vi "DetectHardware.vi"(8 "error in (no error)":errorcluster, 11 "Microscope_RM21 in":refnum<class "Microscope_RM21.lvclass">) -> (0 "error out":errorcluster, 3 "Microscope_RM21 out":refnum<class "Microscope_RM21.lvclass">)   [LabVIEW 2020, in "Microscope_RM21.lvlib" / "Microscope_RM21.lvclass"]
uses:
  Microscope_RM21.lvclass
  D:/Daguan/Development/MMicroscopyFramework/Model/Hardware Abstraction Layer/Microscope/Microscope/Microscope.lvclass
  Stage_MadCityLab/Stage_MadCityLab/Stage_MadCityLab.lvclass
  D:/Daguan/Development/MMicroscopyFramework/Model/Hardware Abstraction Layer/Component/Device/Device/Device.lvclass
  Stage_MadCityLabMicro/Stage_MadCityLabMicro/Stage_MadCityLabMicro.lvclass
  DAQ_QPT_Throlab/DAQ_QPT_Throlab/DAQ_QPT_Throlab.lvclass
  Camera_Prime95B/Camera_Prime95B/Camera_Prime95B.lvclass
  Laser_Oxxius/Laser_Oxxius/Laser_Oxxius.lvclass
  Hardware Abstraction Layer/Microscope/Microscope/Microscope.lvclass
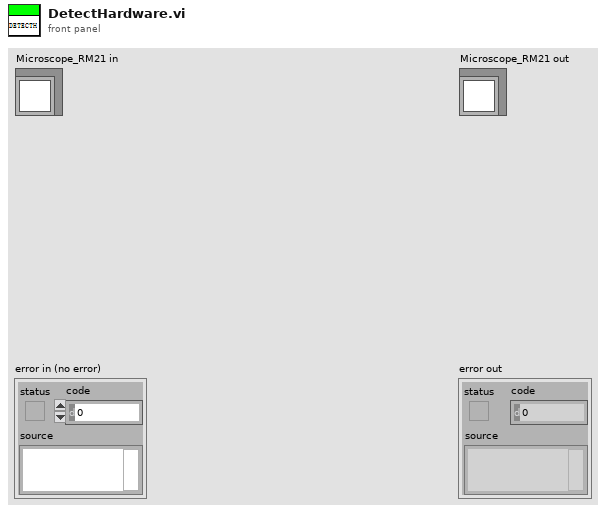
[diagram p1: front panel]
types:
  T1 = cluster{"Label":string, "DeviceType":string, "DefaultDevice? (F)":bool, "StartAcquiring? (F)":bool}
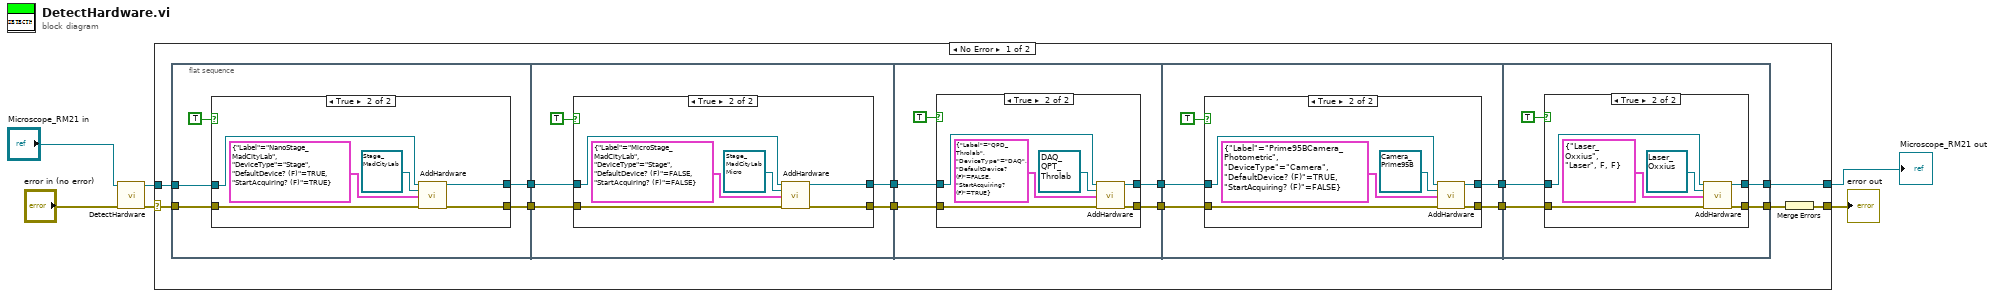
[diagram p0: block diagram]
diagram:
  n1 = call-parent "DetectHardware.vi"("error in (no error)"="error in (no error)", "Microscope in"="Microscope_RM21 in") -> ("error out"=w3:errorcluster, "Microscope out"=w1:refnum<class "Microscope_RM21.lvclass">)  [unwired: 8 in]
  n2 = case shown="No Error" w3 {
    selector: w3 -> [w16 w86]
    tunnel: [w17 w86] -> w5
    tunnel: [w18 w85] -> w6
    tunnel: w1 -> [w7 w85]
    frame No Error {
      n3 = flat-sequence {
        tunnel: [w22] -> w19
        tunnel: w16 -> [w24]
        tunnel: [w23] -> w14
        tunnel: w7 -> [w21]
        tunnel: w19 -> [w37]
        tunnel: [w36] -> w15
        tunnel: w14 -> [w35]
        tunnel: [w34] -> w13
        tunnel: w15 -> [w50]
        tunnel: w13 -> [w48]
        tunnel: [w49] -> w12
        tunnel: [w47] -> w10
        tunnel: w12 -> [w63]
        tunnel: [w60] -> w11
        tunnel: w10 -> [w62]
        tunnel: [w61] -> w9
        tunnel: [w75] -> w18
        tunnel: w11 -> [w76]
        tunnel: w9 -> [w74]
        tunnel: [w73] -> w8
        frame #0 {
          n4 = case shown="True" TRUE {
            tunnel: w24 -> [w25 w32]
            tunnel: [w25 w31] -> w23
            tunnel: [w26 w30] -> w22
            tunnel: w21 -> [w26 w29]
            frame False {
            }
            frame True {
              n5 = call "AddHardware.vi"("Microscope in"=w29, "Device.lvlib:Device.lvclass"=refnum<class "Stage_MadCityLab.lvclass"> refnum ("Stage_MadCityLab.lvlib:Stage_MadCityLab.lvclass"), "Setting"=T1 {"Label"="NanoStage_MadCityLab", "DeviceType"="Stage", "DefaultDevice? (F)"=TRUE, "StartAcquiring? (F)"=TRUE}, "error in (no error)"=w32) -> ("Microscope out"=w30:refnum<class "Microscope_RM21.lvclass">, "error out"=w31:errorcluster)  [unwired: 8 in, 2 out]
            }
          }
        }
        frame #1 {
          n6 = case shown="True" TRUE {
            tunnel: w37 -> [w39 w45]
            tunnel: [w39 w44] -> w36
            tunnel: w35 -> [w38 w43]
            tunnel: [w38 w42] -> w34
            frame False {
            }
            frame True {
              n7 = call "AddHardware.vi"("Microscope in"=w45, "Device.lvlib:Device.lvclass"=refnum<class "Stage_MadCityLabMicro.lvclass"> refnum ("Stage_MadCityLabMicro.lvlib:Stage_MadCityLabMicro.lvclass"), "Setting"=T1 {"Label"="MicroStage_MadCityLab", "DeviceType"="Stage", "DefaultDevice? (F)"=FALSE, "StartAcquiring? (F)"=FALSE}, "error in (no error)"=w43) -> ("Microscope out"=w44:refnum<class "Microscope_RM21.lvclass">, "error out"=w42:errorcluster)  [unwired: 8 in, 2 out]
            }
          }
        }
        frame #2 {
          n8 = case shown="True" TRUE {
            tunnel: w50 -> [w52 w58]
            tunnel: [w52 w57] -> w49
            tunnel: w48 -> [w51 w56]
            tunnel: [w51 w55] -> w47
            frame False {
            }
            frame True {
              n9 = call "AddHardware.vi"("Microscope in"=w58, "Device.lvlib:Device.lvclass"=refnum<class "DAQ_QPT_Throlab.lvclass"> refnum ("DAQ_QPT_Throlab.lvlib:DAQ_QPT_Throlab.lvclass"), "Setting"=T1 {"Label"="QPD_Throlab", "DeviceType"="DAQ", "DefaultDevice? (F)"=FALSE, "StartAcquiring? (F)"=TRUE}, "error in (no error)"=w56) -> ("Microscope out"=w57:refnum<class "Microscope_RM21.lvclass">, "error out"=w55:errorcluster)  [unwired: 8 in, 2 out]
            }
          }
        }
        frame #3 {
          n10 = case shown="True" TRUE {
            tunnel: w63 -> [w65 w71]
            tunnel: w62 -> [w64 w70]
            tunnel: [w64 w69] -> w61
            tunnel: [w65 w68] -> w60
            frame False {
            }
            frame True {
              n11 = call "AddHardware.vi"("Microscope in"=w71, "Device.lvlib:Device.lvclass"=refnum<class "Camera_Prime95B.lvclass"> refnum ("Camera_Prime95B.lvlib:Camera_Prime95B.lvclass"), "Setting"=T1 {"Label"="Prime95BCamera_Photometric", "DeviceType"="Camera", "DefaultDevice? (F)"=TRUE, "StartAcquiring? (F)"=FALSE}, "error in (no error)"=w70) -> ("Microscope out"=w68:refnum<class "Microscope_RM21.lvclass">, "error out"=w69:errorcluster)  [unwired: 8 in, 2 out]
            }
          }
        }
        frame #4 {
          n12 = case shown="True" TRUE {
            tunnel: w76 -> [w78 w84]
            tunnel: [w78 w83] -> w75
            tunnel: w74 -> [w77 w82]
            tunnel: [w77 w81] -> w73
            frame False {
            }
            frame True {
              n13 = call "AddHardware.vi"("Microscope in"=w84, "Device.lvlib:Device.lvclass"=refnum<class "Laser_Oxxius.lvclass"> refnum ("Laser_Oxxius.lvlib:Laser_Oxxius.lvclass"), "Setting"=T1 {"Label"="Laser_Oxxius", "DeviceType"="Laser", "DefaultDevice? (F)"=FALSE, "StartAcquiring? (F)"=FALSE}, "error in (no error)"=w82) -> ("Microscope out"=w83:refnum<class "Microscope_RM21.lvclass">, "error out"=w81:errorcluster)  [unwired: 8 in, 2 out]
            }
          }
        }
      }
      n14 = Merge Errors(w8) -> (w17:errorcluster)
    }
    frame Error {
    }
  }
  "error out" <- w5
  "Microscope_RM21 out" <- w6
